vi "MainDashboard.vi"() -> ()   [LabVIEW 2026]
uses:
  MeasurementCluster.ctl
  SensorCluster.ctl
panel:
  out "Trend":dbl[](graph)
  out "Numeric":i32
  out "Najnowsze rekordy":string[][](table)
  in  "btn_get_history":bool
  in  "btn_load_sensors":bool
  in  "Limit":u16(ring) items=["10", "20", "30", "40", "50"]
  in  "Sensor":string(combo)
  in  "Device":string(combo)
  out "Status API":string
  in  "Clear":bool
  out "History":string[][](table)
  in  "btn_test_api":bool
  in  "refresh":bool
  in  "Auto refresh":bool
  in  "API URL":string
  in  "btn_get_latest":bool
  out "Latest measurement":T1
  in  "stop 2":bool
  out "Trend graph":dbl(graph)
  in  "Interwał":dbl
  in  "stop":bool
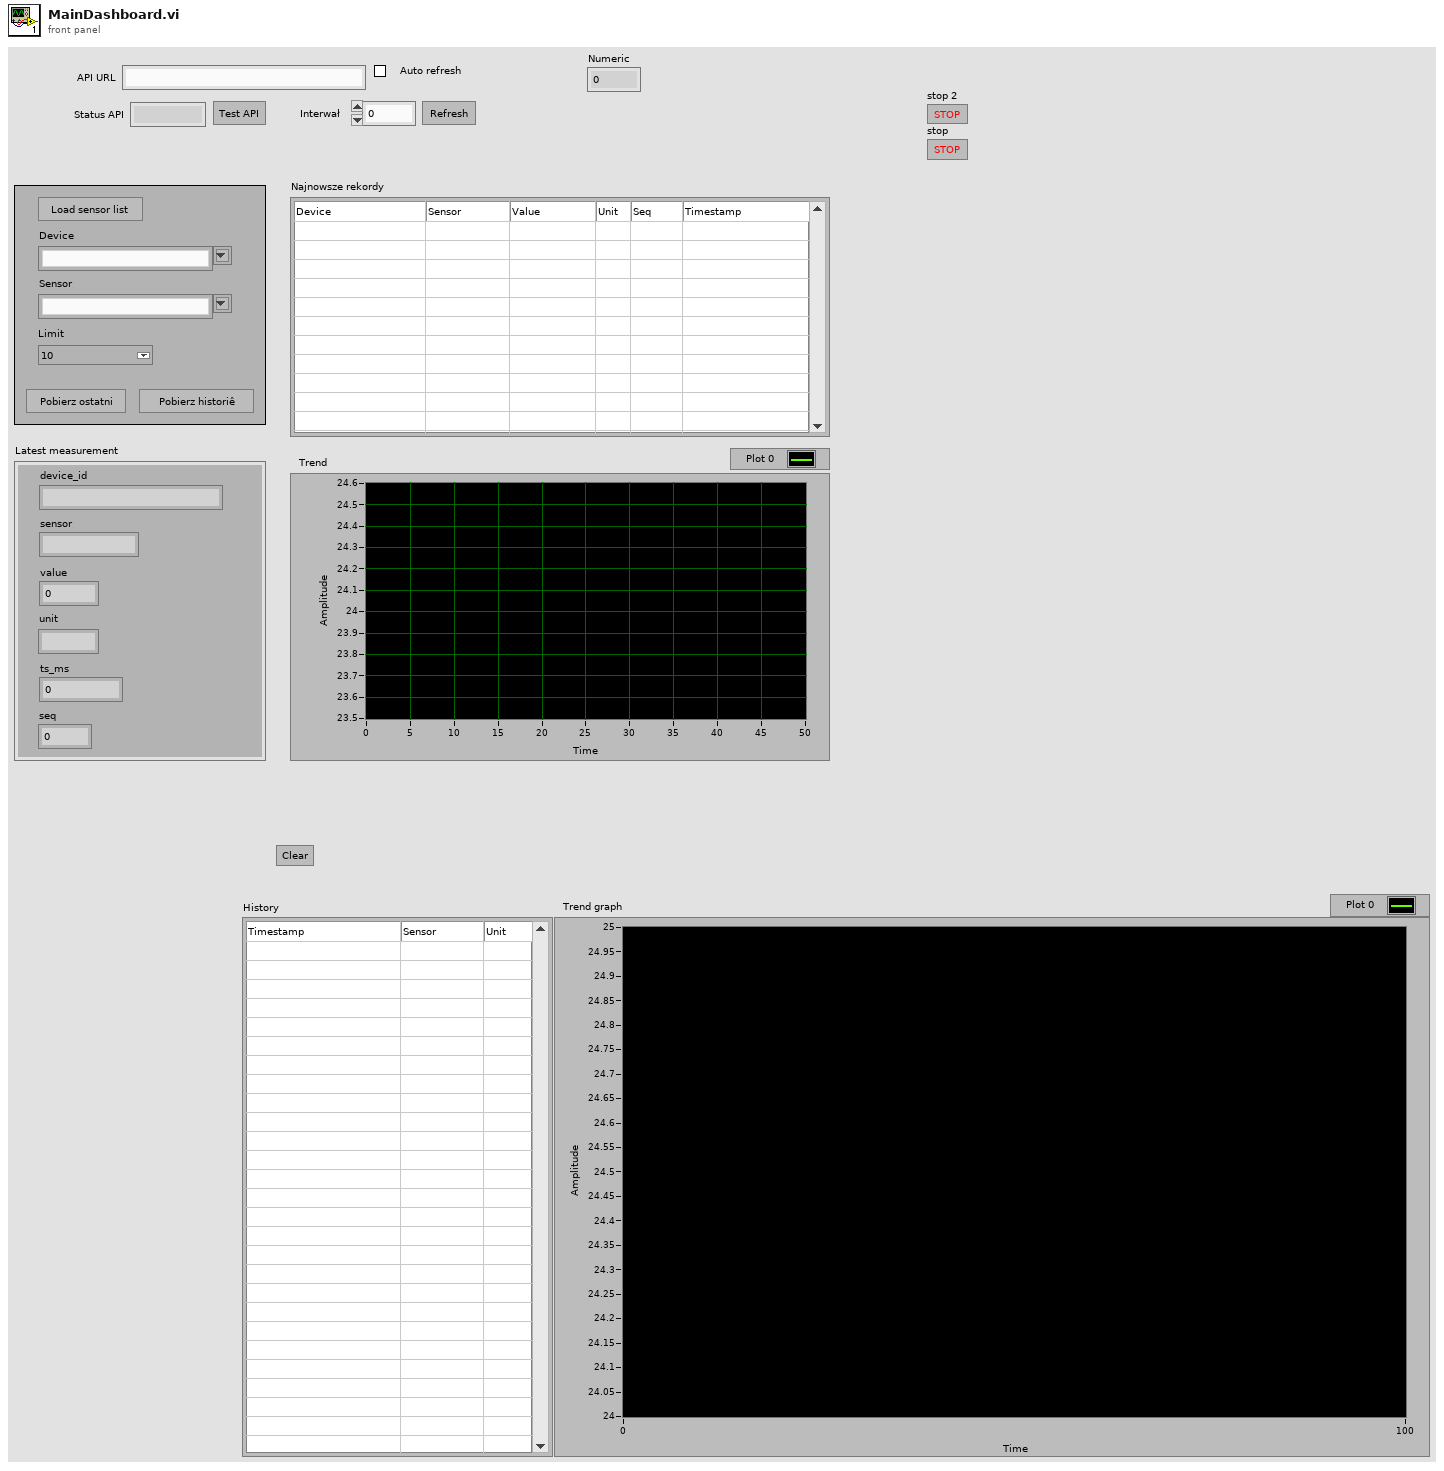
[diagram p1: front panel]
types:
  T1 = typedef "MeasurementCluster.ctl" = cluster{"device_id":string, "sensor":string, "value":dbl, "unit":string, "ts_ms":dbl, "seq":dbl}
  T2 = typedef "SensorCluster.ctl" = cluster{"uuid":string, "name":string, "type":string, "sensor":string, "is_online":bool}
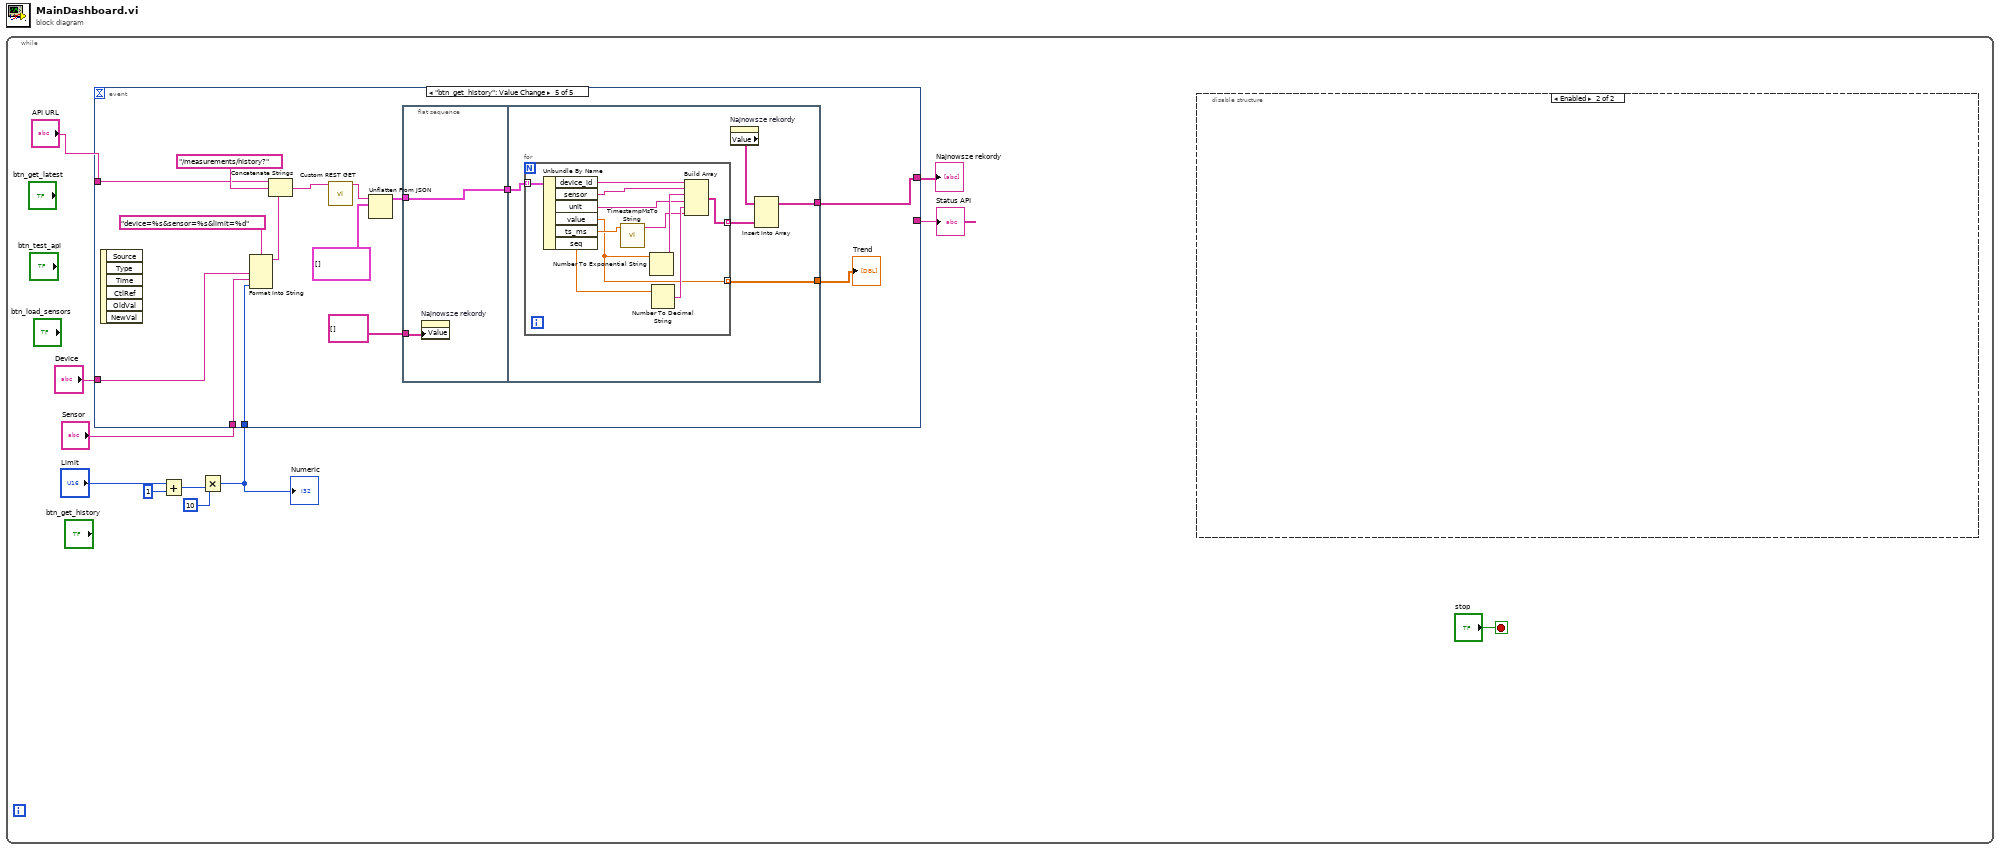
[diagram p0: block diagram]
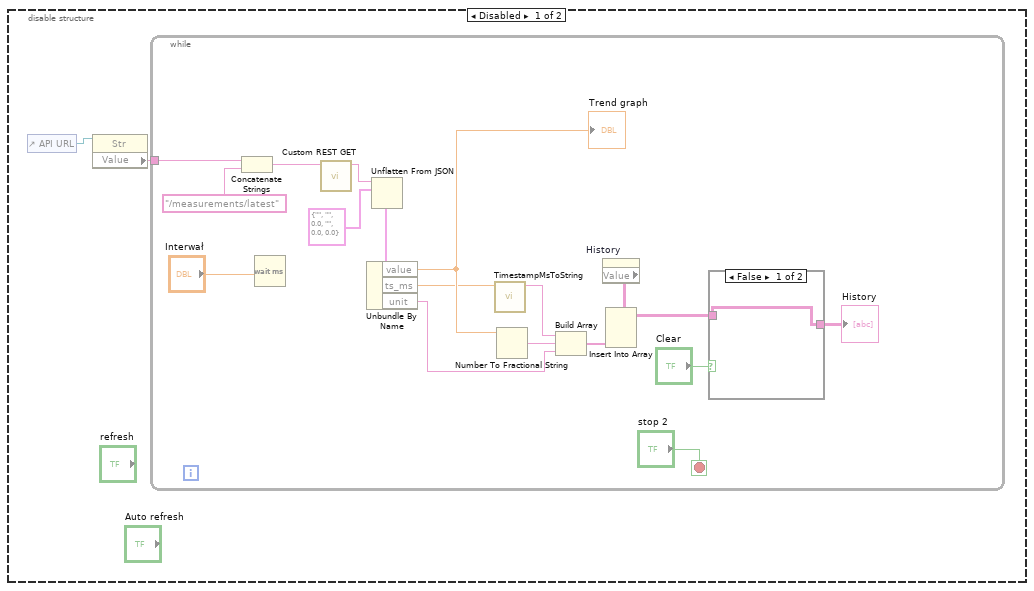
[diagram p2: hidden frame]
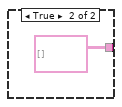
[diagram p3: hidden frame]
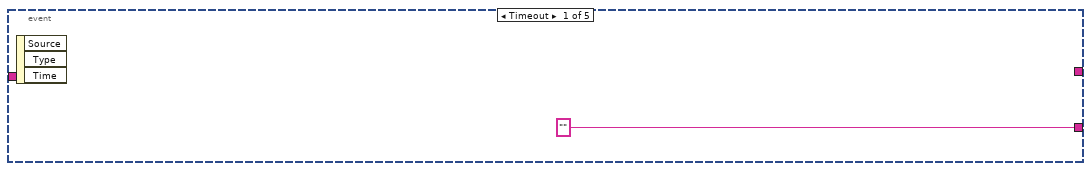
[diagram p4: hidden frame]
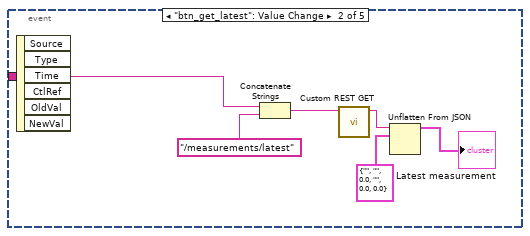
[diagram p5: hidden frame]
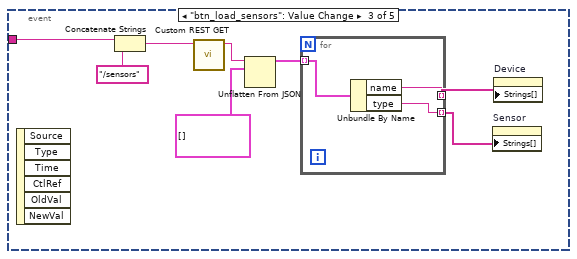
[diagram p6: hidden frame]
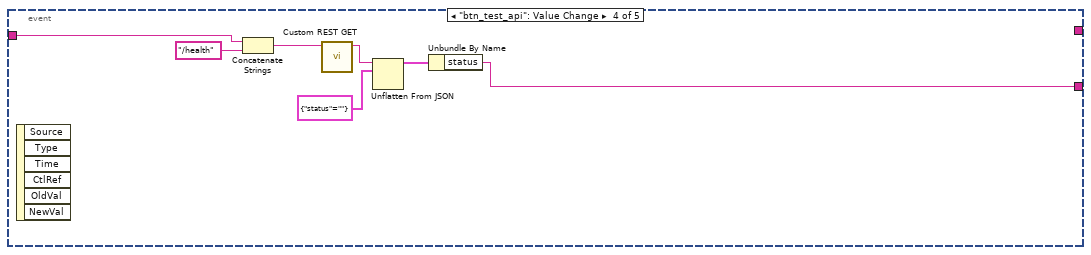
[diagram p7: hidden frame]
diagram:
  n1 = while {
    stop <- "stop" stop-if-true
    n2 = Add(x="Limit", y=u16 1) -> (x+y=w4:u16)
    n3 = Multiply(x=u16 10, y=w4) -> (x*y=w1:u16)
    "Numeric" <- w1
    n4 = event shown="[4] \"btn_get_history\": Value Change" {
      selector: _ -> [_ _ _ _ _]
      dyn-events: _ -> [_ _ _ _ _]
      timeout: _ -> [_ _ _ _ _]
      tunnel: "API URL" -> [_ w37 w45 w53 w70]
      tunnel: ["" ("status") _ _ w52 _] -> w9
      tunnel: "Device" -> [_ _ _ _ w69]
      tunnel: "Sensor" -> [_ _ _ _ w68]
      tunnel: w1 -> [_ _ _ _ w64]
      tunnel: [_ _ _ _ w63] -> w2
      event Timeout {
        n5 = event-data() -> ()  [unwired: 1 in, 3 out]
      }
      event "btn_get_latest": Value Change {
        n6 = event-data() -> ()  [unwired: 1 in, 6 out]
        n7 = Concatenate Strings(w37, "/measurements/latest" ("string")) -> (w39:string)
        n8 = call "Custom REST GET.vi"("Base URL"=w39) -> ("body"=w38:string)  [unwired: 10 in]
        n9 = Unflatten From JSON(JSON string=w38, type and defaults=T1 {"device_id"="", "sensor"="", "value"=0.0, "unit"="", "ts_ms"=0.0, "seq"=0.0} ("Measurement")) -> (value=→"Latest measurement":T1)  [unwired: 5 in, 1 out]
      }
      event "btn_load_sensors": Value Change {
        n10 = event-data() -> ()  [unwired: 1 in, 6 out]
        n11 = Concatenate Strings(w45, "/sensors" ("string")) -> (w47:string)
        n12 = call "Custom REST GET.vi"("Base URL"=w47) -> ("body"=w48:string)  [unwired: 10 in]
        n13 = Unflatten From JSON(JSON string=w48, type and defaults=T2[] []) -> (value=w43:T2[])  [unwired: 5 in, 1 out]
        n14 = for {
          tunnel: w43 -> [w51] mode=indexing
          tunnel: [w50] -> w42 mode=indexing
          tunnel: [w49] -> w41 mode=indexing
          n15 = Unbundle By Name(w51) -> ("name"=w50:string, "type"=w49:string)
        }
        n16 = property on="Sensor" class="CmbBox"("Strings[]"=w41) -> ()  [unwired: 2 in, 2 out]
        n17 = property on="Device" class="CmbBox"("Strings[]"=w42) -> ()  [unwired: 2 in, 2 out]
      }
      event "btn_test_api": Value Change {
        n18 = event-data() -> ()  [unwired: 1 in, 6 out]
        n19 = Concatenate Strings(w53, "/health" ("string")) -> (w56:string)
        n20 = call "Custom REST GET.vi"("Base URL"=w56) -> ("body"=w57:string)  [unwired: 10 in]
        n21 = Unflatten From JSON(JSON string=w57, type and defaults=cluster{"status":string} {"status"=""}) -> (value=w58:cluster{"status":string})  [unwired: 5 in, 1 out]
        n22 = Unbundle By Name(w58) -> ("status"=w52:string)
      }
      event "btn_get_history": Value Change {
        n23 = event-data() -> ()  [unwired: 1 in, 6 out]
        n24 = Format Into String(format string="device=%s&sensor=%s&limit=%d", w69, w68, w64) -> (resulting string=w66:string)  [unwired: 2 in, 1 out]
        n25 = Concatenate Strings(w70, "/measurements/history?" ("string"), w66) -> (w72:string)
        n26 = call "Custom REST GET.vi"("Base URL"=w72) -> ("body"=w73:string)  [unwired: 10 in]
        n27 = Unflatten From JSON(JSON string=w73, type and defaults=T1[] []) -> (value=w61:T1[])  [unwired: 5 in, 1 out]
        n28 = flat-sequence {
          tunnel: [w75] -> w62
          tunnel: w61 -> [w75]
          tunnel: string[][] [] ("Najnowsze rekordy") -> [w74]
          tunnel: [w78] -> w63
          tunnel: w62 -> [w77]
          tunnel: [w76] -> w59
          frame #0 {
            n29 = property on="Najnowsze rekordy" class="Tbl (strict)"("Value"=w74) -> ()  [unwired: 2 in, 2 out]
          }
          frame #1 {
            n30 = for {
              tunnel: [w83] -> w80 mode=indexing
              tunnel: w77 -> [w82] mode=indexing
              tunnel: [w81] -> w76 mode=indexing
              n31 = Unbundle By Name(w82) -> ("device_id"=w91:string, "sensor"=w90:string, "unit"=w84:string, "value"=w81:dbl, "ts_ms"=w86:dbl, "seq"=w88:dbl)
              n32 = call "TimestampMsToString.vi"("timestamp_ms"=w86) -> ("timestamp_str"=w85:string)  [unwired: 10 in]
              n33 = Number To Exponential String(number=w81) -> (E-format string=w89:string)  [unwired: 3 in]
              n34 = Number To Decimal String(number=w88) -> (decimal integer string=w87:string)  [unwired: 1 in]
              n35 = Build Array(w91, w90, w89, w84, w87, w85) -> (w83:string[])
            }
            n36 = property on="Najnowsze rekordy" class="Tbl (strict)"() -> ("Value"=w79:string[][])  [unwired: 2 in, 2 out]
            n37 = Insert Into Array(array=w79, new element=w80) -> (w78:string[][])  [unwired: 2 in]
          }
        }
        "Trend" <- w59
      }
    }
    "Status API" <- w9
    "Najnowsze rekordy" <- w2
    n38 = disable-structure shown="Enabled" {
      frame Disabled {
        n39 = control-ref of="API URL"() -> (w13:refnum<vi>)
        n40 = property class="Str"(reference=w13) -> ("Value"=w12:string)  [unwired: 1 in, 2 out]
        n41 = while {
          tunnel: w12 -> [w28]
          stop <- "stop 2" stop-if-true
          n42 = Concatenate Strings(w28, "/measurements/latest" ("string")) -> (w31:string)
          n43 = Wait (ms)(milliseconds to wait="Interwał") -> ()  [unwired: 1 out]
          n44 = call "Custom REST GET.vi"("Base URL"=w31) -> ("body"=w30:string)  [unwired: 10 in]
          n45 = Unflatten From JSON(JSON string=w30, type and defaults=T1 {"device_id"="", "sensor"="", "value"=0.0, "unit"="", "ts_ms"=0.0, "seq"=0.0} ("Measurement")) -> (value=w26:T1)  [unwired: 5 in, 1 out]
          n46 = Unbundle By Name(w26) -> ("value"=w23:dbl, "ts_ms"=w16:dbl, "unit"=w20:string)
          "Trend graph" <- w23
          n47 = call "TimestampMsToString.vi"("timestamp_ms"=w16) -> ("timestamp_str"=w15:string)  [unwired: 10 in]
          n48 = Number To Fractional String(number=w23) -> (F-format string=w22:string)  [unwired: 3 in]
          n49 = Build Array(w15, w22, w20) -> (w21:string[])
          n50 = property on="History" class="Tbl (strict)"() -> ("Value"=w24:string[][])  [unwired: 2 in, 2 out]
          n51 = Insert Into Array(array=w24, new element=w21) -> (w18:string[][])  [unwired: 2 in]
          n52 = case shown="False" "Clear" {
            tunnel: [w32 string[][] [] ("Value")] -> w17
            tunnel: w18 -> [w32 _]
            frame False {
            }
            frame True {
            }
          }
          "History" <- w17
        }
      }
      frame Enabled {
      }
    }
  }
